vi "case_default_zero.vi"(11 "selector":i32) -> (3 "result":i32=20)   [LabVIEW 2020]
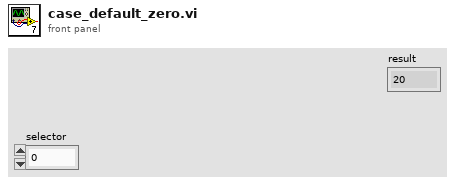
[diagram p1: front panel]
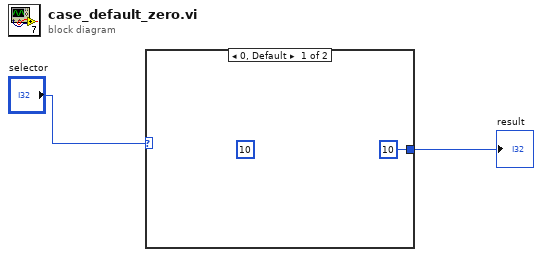
[diagram p0: block diagram]
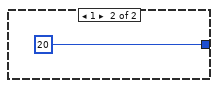
[diagram p2: hidden frame]
diagram:
  n1 = case shown="0, Default" "selector" {
    tunnel: [10 20] -> w1
    frame 0, Default {
      (unwired) 10
    }
    frame 1 {
    }
  }
  "result" <- w1
